vi "uniqueLineForOneRobot.vi"(11 "Robot in":refnum<class "Robot.lvclass">) -> (3 "Robot out":refnum<class "Robot.lvclass">)   [LabVIEW 2020, in "Game.lvclass"]
uses:
  Game.lvclass
  Robot_class/Robot.lvclass
  C:/RoboIME/SSL_AI/Object_class/Object.lvclass
  Object_class/Object.lvclass/Object.ctl
  Robot_class/Robot.lvclass/Robot.ctl
  Object_class/Read x.vi
  Object_class/Read y.vi
  Robot_class/Read dest_x.vi
  Robot_class/Read dest_y.vi
  Robot_class/Write path.vi
  Robot_class/Write path_smooth.vi
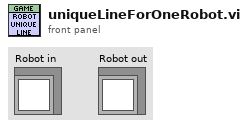
[diagram p1: front panel]
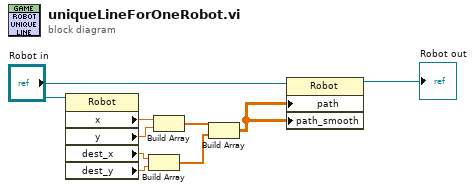
[diagram p0: block diagram]
diagram:
  n1 = property class="Robot"(reference="Robot in") -> ("x"=w3:dbl, "y"=w4:dbl, "dest_x"=w5:dbl, "dest_y"=w6:dbl)  [unwired: 1 in, 2 out]
  n2 = Build Array(w5, w6) -> (w8:dbl[])
  n3 = Build Array(w3, w4) -> (w7:dbl[])
  n4 = Build Array(w7, w8) -> (w9:dbl[][])
  n5 = property class="Robot"(reference="Robot in", "path"=w9, "path_smooth"=w9) -> (reference out=→"Robot out":refnum<class "Robot.lvclass">)  [unwired: 1 in, 1 out]
